vi "Create 986x Support.vi"(8 "error in (no error)":errorcluster, 10 "986x Support":T2, 11 "Device Item Ref in":T1 format="%.0x") -> (0 "error out":errorcluster, 3 "Device Ref out":T1 format="%.0x")   [LabVIEW 2015, in "Diagnostics Addon System Explorer.lvlib"]
uses:
  System Explorer/Diagnostics Addon System Explorer.lvlib
  <vilib>/NI Veristand/Custom Device API/Custom Device Item Ref.ctl
  Exported 986x Support.ctl
  <vilib>/NI Veristand/Custom Device API/Set Item Property (U16).vi
  <vilib>/NI Veristand/Custom Device API/Set Item Property (Path).vi
  GUID Lookup.vi
  <vilib>/NI Veristand/Custom Device API/Set Item Property (Boolean).vi
  Diagnostics Addon Shared.lvlib
  <vilib>/NI Veristand/Custom Device API/Custom Device API.lvlib
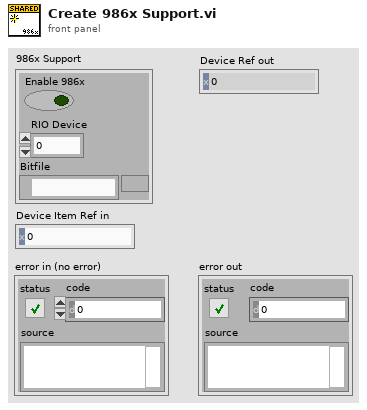
[diagram p1: front panel]
types:
  T1 = typedef "Custom Device API.lvlib/Custom Device Item Ref.ctl" = u64
  T2 = typedef "Diagnostics Addon System Explorer.lvlib/Exported 986x Support.ctl" = cluster{"Enable 986x":bool, "RIO Device":u16, "Bitfile":path}
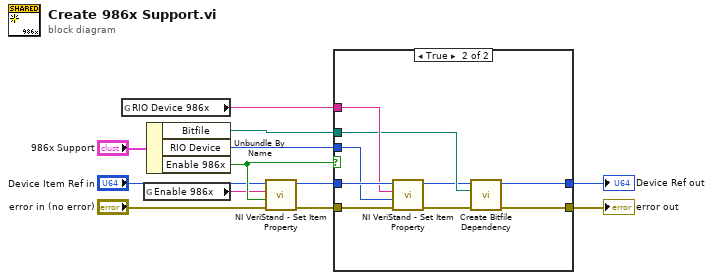
[diagram p0: block diagram]
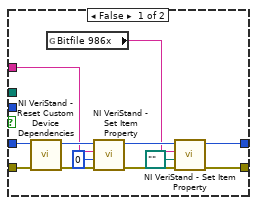
[diagram p2: hidden frame]
diagram:
  n1 = global read "GUID Lookup.vi" "RIO Device 986x"() -> (w11:string)
  n2 = global read "GUID Lookup.vi" "Enable 986x"() -> (w1:string)
  n3 = Unbundle By Name("986x Support") -> ("Bitfile"=w12:path, "RIO Device"=w10:u16, "Enable 986x"=w9:bool)
  n4 = call-poly <vilib>:"NI VeriStand - Set Item Property.vi"("error in (no error)"="error in (no error)", "Value"=w9, "Property Name"=w1, "Item Ref in"="Device Item Ref in") -> ("error out"=w5:errorcluster, "Item Ref out"=w7:T1)  [unwired: 5 in, 1 out]
  n5 = case shown="True" w9 {
    tunnel: w5 -> [w24 w33]
    tunnel: [w20 w28] -> w6
    tunnel: w7 -> [w23 w32]
    tunnel: w11 -> [w17 w30]
    tunnel: [w14 w25] -> w8
    tunnel: w10 -> [_ w31]
    tunnel: w12 -> [_ w27]
    frame False {
      n6 = call <vilib>:"NI VeriStand - Reset Custom Device Dependencies.vi"("error in (no error)"=w24, "Device Ref in"=w23) -> ("error out"=w21:errorcluster, "Device Ref out"=w19:T1)  [unwired: 8 in]
      n7 = global read "GUID Lookup.vi" "Bitfile 986x"() -> (w13:string)
      n8 = call-poly <vilib>:"NI VeriStand - Set Item Property.vi"("error in (no error)"=w21, "Value"=u16 0, "Property Name"=w17, "Item Ref in"=w19) -> ("error out"=w22:errorcluster, "Item Ref out"=w18:T1)  [unwired: 5 in, 1 out]
      n9 = call-poly <vilib>:"NI VeriStand - Set Item Property.vi"("error in (no error)"=w22, "Value"=path "", "Property Name"=w13, "Item Ref in"=w18) -> ("error out"=w20:errorcluster, "Item Ref out"=w14:T1)  [unwired: 5 in, 1 out]
    }
    frame True {
      n10 = call-poly <vilib>:"NI VeriStand - Set Item Property.vi"("error in (no error)"=w33, "Value"=w31, "Property Name"=w30, "Item Ref in"=w32) -> ("error out"=w29:errorcluster, "Item Ref out"=w26:T1)  [unwired: 5 in, 1 out]
      n11 = call "Create Bitfile Dependency.vi"("error in (no error)"=w29, "Bitfile Path"=w27, "Item Ref in"=w26) -> ("error out"=w28:errorcluster, "Device Ref out"=w25:T1)  [unwired: 7 in]
    }
  }
  "Device Ref out" <- w8
  "error out" <- w6
